vi "lv-ros-bridge.vi"(8 "error in (no error)":errorcluster, 9 "subscribe message":string="{ \"op\": \"subscribe\", \"topic\" : \"/chatter_joy\" }", 10 "rosbridge port":u16=9090, 11 "rosbridge server IP":string="192.168.5.103") -> (0 "error out":errorcluster, 2 "axes":sgl[](array[numeric]), 3 "buttons":i32[](array[numeric]))   [LabVIEW 2013]
uses:
  <vilib>/Intelligent Energy/WebSockets API/WebSockets/WebSockets.lvlib
panel:
  in  "advertise message":string
  out "output cluster":T1
  in  "msg.vel5":i16
  in  "msg.vel4":i16
  in  "msg.vel3":i16
  in  "msg.vel2":i16
  in  "msg.vel1":i16
  in  "msg.vel0":i16
  in  "Topic to write":string
  in  "outgoing message":T1
  out "incomming\nmessage":T2
  out "value":T2
  in  "?":T2
  out "raw frame":string
  in  "stop":bool
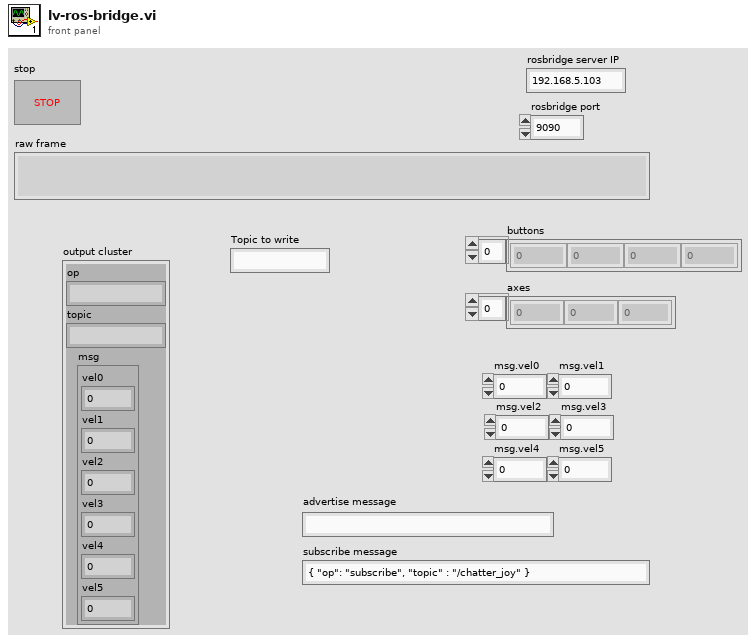
[diagram p1: front panel]
types:
  T1 = cluster{"op":string, "topic":string, "msg":cluster{"vel0":i16, "vel1":i16, "vel2":i16, "vel3":i16, "vel4":i16, "vel5":i16}}
  T2 = cluster{"topic":string, "msg":cluster{"header":cluster{"seq":u32, "stamp":cluster{"secs":u32, "nsecs":i32}, "frame_id":string}, "buttons":i32[], "axes":sgl[]}, "op":string}
  T3 = cluster{"header":cluster{"seq":u32, "stamp":cluster{"secs":u32, "nsecs":i32}, "frame_id":string}, "buttons":i32[], "axes":sgl[]}
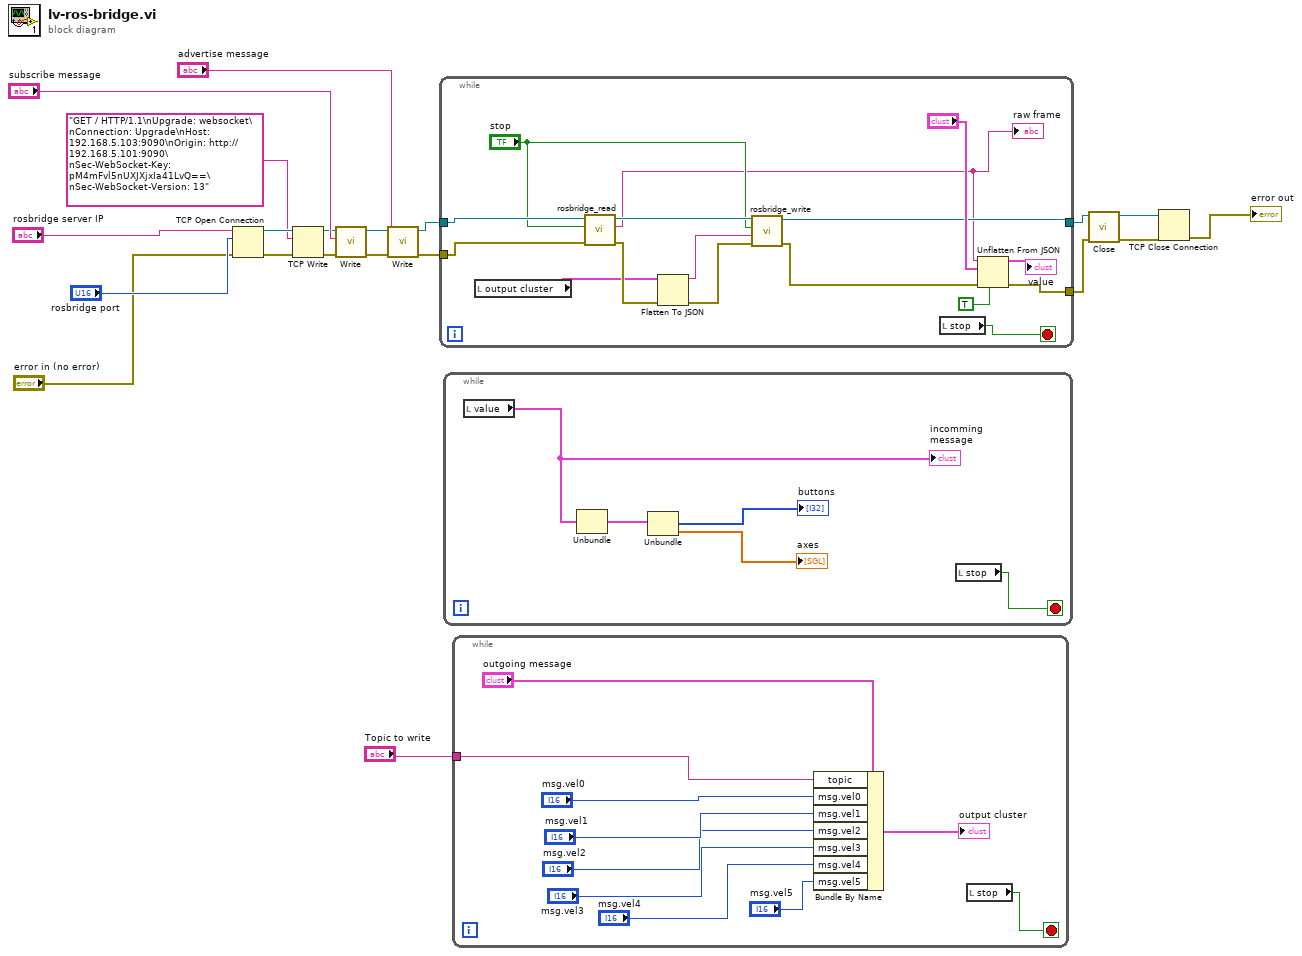
[diagram p0: block diagram]
diagram:
  n1 = TCP Open Connection(address="rosbridge server IP", remote port or service name="rosbridge port", error in (no error)="error in (no error)") -> (connection ID=w18:refnum<k5>, error out=w16:errorcluster)  [unwired: 2 in]
  n2 = TCP Write(connection ID=w18, data in="GET / HTTP/1.1\nUpgrade: websocket\nConnection: Upgrade\nHost: 192.168.5.103:9090\nOrigin: http://192.168.5.101:9090\nSec-WebSocket-Key: pM4mFvl5nUXJXjxIa41LvQ==\nSec-WebSocket-Version: 13", error in (no error)=w16) -> (connection ID out=w12:refnum<k5>, error out=w11:errorcluster)  [unwired: 1 in, 1 out]
  n3 = call <vilib>:"Write.vi"("error in (no error)"=w11, "Data"="subscribe message", "WebSocket Connection in"=w12) -> ("error out"=w4:errorcluster, "WebSocket Connection out"=w5:refnum<k5>)  [unwired: 7 in]
  n4 = call <vilib>:"Write.vi"("error in (no error)"=w4, "Data"="advertise message", "WebSocket Connection in"=w5) -> ("error out"=w3:errorcluster, "WebSocket Connection out"=w2:refnum<k5>)  [unwired: 7 in]
  n5 = while {
    tunnel: [w30] -> w10
    tunnel: [w36] -> w9
    tunnel: w2 -> [w29]
    tunnel: w3 -> [w22]
    stop <- w32 stop-if-true
    n6 = local read "output cluster"() -> (w23:T1)
    n7 = call "rosbridge_read.vi"("error in (no error)"=w22, "stop"="stop", "TCP Network Connection in"=w29) -> ("error out"=w26:errorcluster, "String"=w21:string, "TCP Network Connection out"=w28:refnum<k5>)  [unwired: 6 in]
    "raw frame" <- w21
    n8 = Flatten To JSON(anything=w23, error in (no error)=w26) -> (JSON string=w24:string, 11:w25:errorcluster)  [unwired: 1 in]
    n9 = call "rosbridge_write.vi"("error in (no error)"=w25, "JSON string"=w24, "stop"="stop", "TCP Network Connection in"=w28) -> ("error out"=w31:errorcluster, "TCP Network Connection out"=w30:refnum<k5>)  [unwired: 6 in]
    n10 = local read "stop"() -> (w32:bool)
    n11 = Unflatten From JSON(JSON string=w21, type and defaults="?", default null elements? (F)=TRUE, error in (no error)=w31) -> (value=→"value":T2, error out=w36:errorcluster)  [unwired: 3 in]
  }
  n12 = while {
    stop <- w37 stop-if-true
    n13 = local read "value"() -> (w41:T2)
    "incomming\nmessage" <- w41
    n14 = Unbundle(w41) -> ("msg"=w40:T3)  [unwired: 2 out]
    n15 = Unbundle(w40) -> ("buttons"=→"buttons":i32[], "axes"=→"axes":sgl[])  [unwired: 1 out]
    n16 = local read "stop"() -> (w37:bool)
  }
  n17 = while {
    tunnel: "Topic to write" -> [w50]
    stop <- w42 stop-if-true
    n18 = Bundle By Name(cluster="outgoing message", "topic"=w50, "msg.vel0"="msg.vel0", "msg.vel1"="msg.vel1", "msg.vel2"="msg.vel2", "msg.vel3"="msg.vel3", "msg.vel4"="msg.vel4", "msg.vel5"="msg.vel5") -> (→"output cluster":T1)
    n19 = local read "stop"() -> (w42:bool)
  }
  n20 = call <vilib>:"Close.vi"("error in (no error)"=w9, "WebSocket Connection in"=w10) -> ("error out"=w13:errorcluster, "WebSocket Connection in"=w14:refnum<k5>)  [unwired: 8 in]
  n21 = TCP Close Connection(connection ID=w14, error in (no error)=w13) -> (error out=→"error out":errorcluster)  [unwired: 1 in, 1 out]
